vi "_AllThingsGazebo.vi"   [LabVIEW 2012]
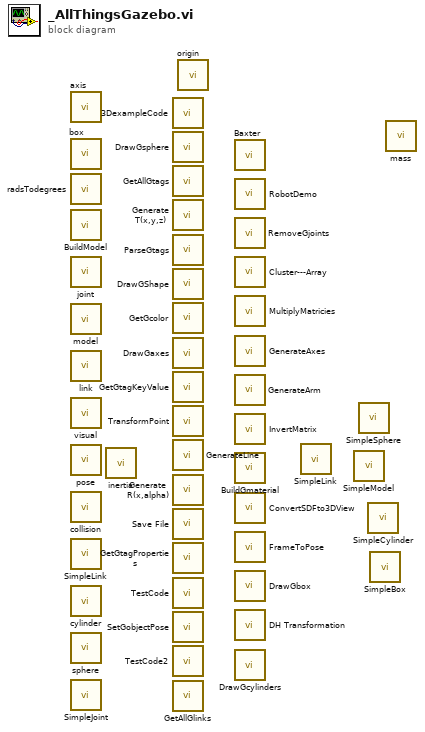
[diagram p0: block diagram]
diagram:
  n1 = call <userlib>:"axis.vi"() -> ()  [unwired: 4 in, 1 out]
  n2 = call <userlib>:"box.vi"() -> ()  [unwired: 4 in, 1 out]
  n3 = call <userlib>:"radsTodegrees.vi"() -> ()  [unwired: 1 in, 1 out]
  n4 = call <userlib>:"BuildModel.vi"() -> ()  [unwired: 4 in, 2 out]
  n5 = call <userlib>:"joint.vi"() -> ()  [unwired: 4 in, 1 out]
  n6 = call <userlib>:"model.vi"() -> ()  [unwired: 4 in, 1 out]
  n7 = call <userlib>:"link.vi"() -> ()  [unwired: 4 in, 1 out]
  n8 = call <userlib>:"visual.vi"() -> ()  [unwired: 4 in, 1 out]
  n9 = call <userlib>:"pose.vi"() -> ()  [unwired: 4 in, 1 out]
  n10 = call <userlib>:"collision.vi"() -> ()  [unwired: 4 in, 1 out]
  n11 = call <userlib>:"SimpleLink.vi"() -> ()  [unwired: 6 in, 1 out]
  n12 = call <userlib>:"cylinder.vi"() -> ()  [unwired: 4 in, 1 out]
  n13 = call <userlib>:"sphere.vi"() -> ()  [unwired: 4 in, 1 out]
  n14 = call <userlib>:"SimpleJoint.vi"() -> ()  [unwired: 5 in, 1 out]
  n15 = call <userlib>:"inertia.vi"() -> ()  [unwired: 4 in, 1 out]
  n16 = call <userlib>:"3DexampleCode.vi"() -> ()  [unwired: 12 in]
  n17 = call <userlib>:"DrawGsphere.vi"() -> ()  [unwired: 3 in, 2 out]
  n18 = call <userlib>:"GetAllGtags.vi"() -> ()  [unwired: 2 in, 3 out]
  n19 = call <userlib>:"Generate T(x,y,z).vi"() -> ()  [unwired: 3 in, 1 out]
  n20 = call <userlib>:"ParseGtags.vi"() -> ()  [unwired: 2 in, 4 out]
  n21 = call <userlib>:"DrawGShape.vi"() -> ()  [unwired: 2 in, 2 out]
  n22 = call <userlib>:"GetGcolor.vi"() -> ()  [unwired: 1 in, 2 out]
  n23 = call <userlib>:"DrawGaxes.vi"() -> ()  [unwired: 2 in, 1 out]
  n24 = call <userlib>:"GetGtagKeyValue.vi"() -> ()  [unwired: 2 in, 1 out]
  n25 = call <userlib>:"TransformPoint.vi"() -> ()  [unwired: 2 in, 2 out]
  n26 = call <userlib>:"GenerateLine.vi"() -> ()  [unwired: 4 in, 1 out]
  n27 = call <userlib>:"Generate R(x,alpha).vi"() -> ()  [unwired: 3 in, 1 out]
  n28 = call <userlib>:"Save File.vi"() -> ()  [unwired: 3 in, 1 out]
  n29 = call <userlib>:"GetGtagProperties.vi"() -> ()  [unwired: 1 in, 1 out]
  n30 = call <userlib>:"TestCode.vi"() -> ()  [unwired: 1 in]
  n31 = call <userlib>:"SetGobjectPose.vi"() -> ()  [unwired: 2 in, 2 out]
  n32 = call <userlib>:"TestCode2.vi"() -> ()  [unwired: 1 in]
  n33 = call <userlib>:"GetAllGlinks.vi"() -> ()  [unwired: 2 in, 2 out]
  n34 = call <userlib>:"origin.vi"() -> ()  [unwired: 1 in, 1 out]
  n35 = call <userlib>:"Baxter.vi"() -> ()  [unwired: 12 in]
  n36 = call <userlib>:"RobotDemo.vi"() -> ()  [unwired: 12 in]
  n37 = call <userlib>:"RemoveGjoints.vi"() -> ()  [unwired: 1 in, 1 out]
  n38 = call <userlib>:"Cluster---Array.vi"() -> ()  [unwired: 2 in, 2 out]
  n39 = call <userlib>:"MultiplyMatricies.vi"() -> ()  [unwired: 2 in, 2 out]
  n40 = call <userlib>:"GenerateAxes.vi"() -> ()  [unwired: 6 in, 1 out]
  n41 = call <userlib>:"GenerateArm.vi"() -> ()  [unwired: 5 in, 1 out]
  n42 = call <userlib>:"InvertMatrix.vi"() -> ()  [unwired: 2 in, 2 out]
  n43 = call <userlib>:"BuildGmaterial.vi"() -> ()  [unwired: 2 in, 1 out]
  n44 = call <userlib>:"ConvertSDFto3DView.vi"() -> ()  [unwired: 2 in, 2 out]
  n45 = call <userlib>:"FrameToPose.vi"() -> ()  [unwired: 1 in, 1 out]
  n46 = call <userlib>:"DrawGbox.vi"() -> ()  [unwired: 3 in, 2 out]
  n47 = call <userlib>:"DH Transformation.vi"() -> ()  [unwired: 3 in, 1 out]
  n48 = call <userlib>:"DrawGcylinders.vi"() -> ()  [unwired: 3 in, 2 out]
  n49 = call <userlib>:"SimpleLink.vi"() -> ()  [unwired: 6 in, 1 out]
  n50 = call <userlib>:"SimpleModel.vi"() -> ()  [unwired: 4 in, 1 out]
  n51 = call <userlib>:"SimpleSphere.vi"() -> ()  [unwired: 6 in, 1 out]
  n52 = call <userlib>:"SimpleCylinder.vi"() -> ()  [unwired: 6 in, 1 out]
  n53 = call <userlib>:"SimpleBox.vi"() -> ()  [unwired: 6 in, 1 out]
  n54 = call <userlib>:"mass.vi"() -> ()  [unwired: 1 in, 1 out]
